vi "Write Error Log.vi"(8 "error in (no error)":errorcluster, 10 "Error Log":path, 11 "Error in":refnum<class "Error.lvclass">) -> (0 "error out":errorcluster, 3 "Error out":refnum<class "Error.lvclass">)   [LabVIEW 2019, in "TSC Error.lvlib" / "Error.lvclass"]
doc: "Data Member Access to write the location of the error log.\n\nInputs:\n-Error in [obj] - the dynamic dispatch input class\n-Error Log [path] - the data member access input\n-error in\n\nOutputs:\n-Error out [obj] - the dynamic dispatch output class\n-error out\n________________________________________________________________________________\n<b>Code Developed By:</b>\nDaniel Coons\nTechnology Service Corporation\n1983 S Liberty Drive\nBloomington, IN 47403\nPhone: 812 558-7100\ndaniel.coons@tsc.com\nwww.tsc.com\n\n<b>Date Created:</b> 04 APR 2016\n<b>Date Updated:</b>"
uses:
  Error.lvclass
  Error.lvclass/Error.ctl
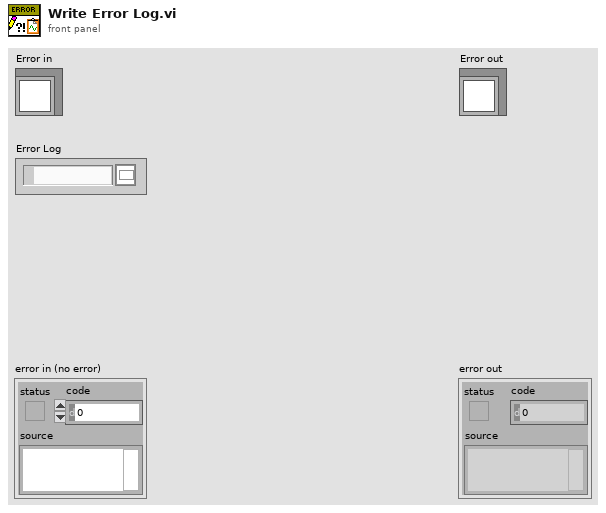
[diagram p1: front panel]
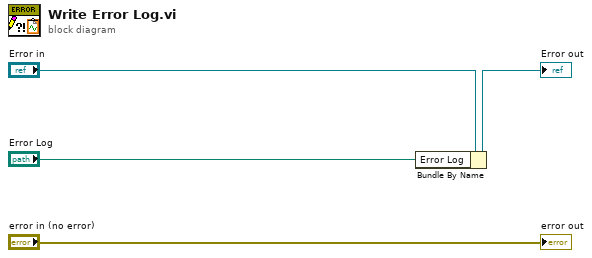
[diagram p0: block diagram]
diagram:
  n1 = Bundle By Name(cluster="Error in", "Error Log"="Error Log") -> (→"Error out":refnum<class "Error.lvclass">)
  "error out" <- "error in (no error)"
